vi "RunningAverage-RemoveResultChannel.vi"(8 "Error in":errorcluster, 11 "Custom Device ref":T1 format="%.0x") -> (0 "Error out":errorcluster, 3 "Custom Device ref out":T1 format="%.0x")   [LabVIEW 2017, in "Waveform-Processing-Custom-Device Shared.lvlib" / "Running Average.lvlib"]
doc: "This application uses the Result Section group to find and remove output channel of the \"RMS\" channel type"
uses:
  Running Average.lvlib
  <vilib>/NI Veristand/Custom Device API/Custom Device Item Ref.ctl
  Constants.vi
  <vilib>/NI Veristand/Custom Device API/Get Item Property (Dependent Node Pointer).vi
  System Explorer/Waveform-Processing-Custom-Device System Explorer.lvlib
  <vilib>/NI VeriStand/Custom Device API/Custom Device API.lvlib
  Waveform-Processing-Custom-Device Shared.lvlib
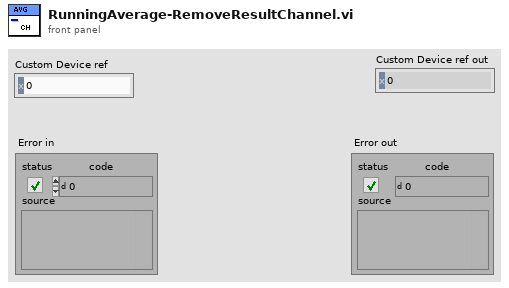
[diagram p1: front panel]
types:
  T1 = typedef "Custom Device API.lvlib/Custom Device Item Ref.ctl" = u64
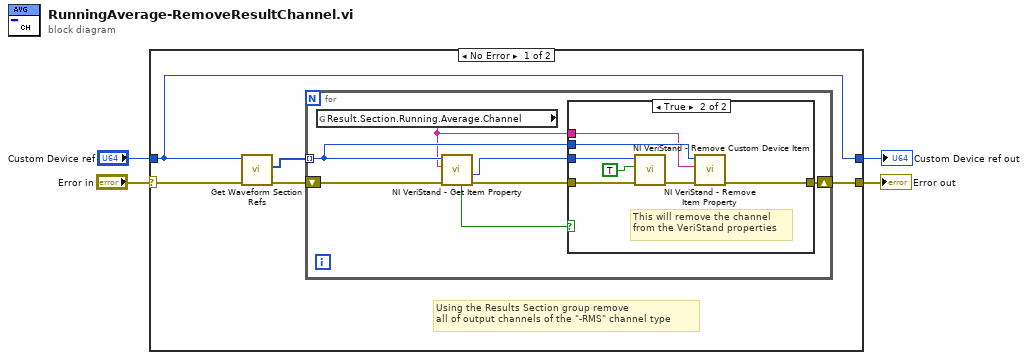
[diagram p0: block diagram]
diagram:
  n1 = case shown="No Error" "Error in" {
    selector: "Error in" -> [w7 w26]
    tunnel: "Custom Device ref" -> [w5 w25]
    tunnel: [w8 w26] -> w3
    tunnel: [w5 w25] -> w1
    frame No Error {
      # "Using the Results Section group remove \nall of output channels of the \"-RMS\" channel type"
      n2 = call "Get Waveform Section Refs.vi"("Error in"=w7, "Device Ref in"=w5) -> ("Error out"=w9:errorcluster, "Result Section Refs"=w6:T1[])  [unwired: 7 in, 1 out]
      n3 = for {
        tunnel: w6 -> [w11] mode=indexing
        shift-right: [w14] -> w8
        shift-left: w9 -> [w16]
        n4 = global read "Constants.vi" "Result.Section.Running.Average.Channel"() -> (w10:string)
        n5 = call-poly <vilib>:"NI VeriStand - Get Item Property.vi"("error in (no error)"=w16, "Property Name"=w10, "Item Ref in"=w11) -> ("error out"=w15:errorcluster, "Dependent Node Ref"=w13:T1, "Found"=w12:bool)  [unwired: 5 in, 1 out]
        n6 = case shown="True" w12 {
          tunnel: w15 -> [w17 w23]
          tunnel: [w17 w21] -> w14
          tunnel: w13 -> [_ w20]
          tunnel: w11 -> [_ w19]
          tunnel: w10 -> [_ w18]
          frame False {
          }
          frame True {
            # "This will remove the channel \nfrom the VeriStand properties"
            n7 = call <vilib>:"NI VeriStand - Remove Custom Device Item.vi"("error in (no error)"=w23, "Force Delete (F)"=TRUE, "Item Ref in"=w20) -> ("error out"=w22:errorcluster)  [unwired: 7 in, 1 out]
            n8 = call <vilib>:"NI VeriStand - Remove Item Property.vi"("error in (no error)"=w22, "Property Name"=w18, "Item Ref in"=w19) -> ("error out"=w21:errorcluster)  [unwired: 6 in, 2 out]
          }
        }
      }
    }
    frame Error {
    }
  }
  "Error out" <- w3
  "Custom Device ref out" <- w1
